vi "lp-server-timeouts.vi"() -> ()   [LabVIEW 2014]
uses:
  lvnanomsg/nanomsg_context.lvclass
  lvnanomsg/nanomsg_socket.lvclass
panel:
  in  "stop?":bool
  out "loop":i32
  in  "timeout":u32=500
  in  "endpoint":string="tcp://127.0.0.1:5555"
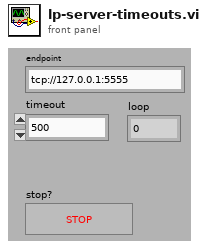
[diagram p1: front panel]
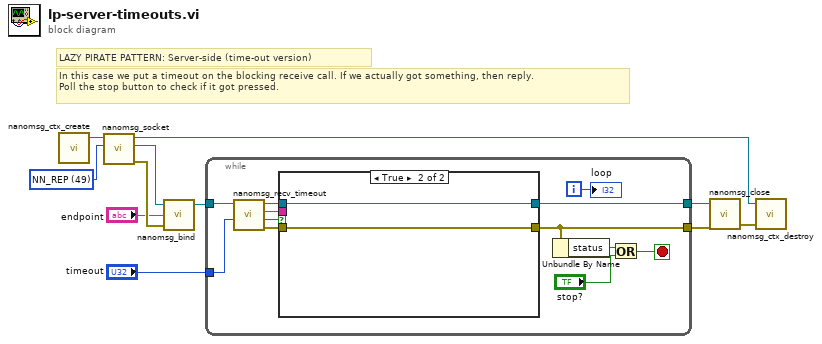
[diagram p0: block diagram]
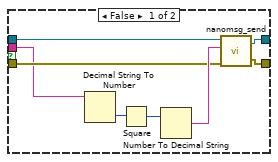
[diagram p2: hidden frame]
diagram:
  w7 = 49 items=["NN_WS"=-4, "NN_TCP"=-3, "NN_IPC"=-2, "NN_INPROC"=-1, "NN_SOL_SOCKET"=0, "NN_PAIR"=16, "NN_PUB"=32, "NN_SUB"=33, "NN_REQ"=48, "NN_REP"=49, "NN_PUSH"=80, "NN_PULL"=81, "NN_SURVEYOR"=98, "NN_RESPONDENT"=99, "NN_BUS"=112] ("socket type")
  # "In this case we put a timeout on the blocking receive call. If we actually got something, then reply.\nPoll the stop button to check if it got pressed."
  # "LAZY PIRATE PATTERN: Server-side (time-out version)"
  n1 = call "nanomsg_ctx_create.vi"() -> ("context out"=w6:refnum<class "nanomsg_context.lvclass">)  [unwired: 4 in, 1 out]
  n2 = call "nanomsg_socket.vi"("socket type"=w7, "context in"=w6) -> ("error out"=w10:errorcluster, "socket out"=w2:refnum<class "nanomsg_socket.lvclass">, "context out"=w1:refnum<class "nanomsg_context.lvclass">)  [unwired: 3 in]
  n3 = call "nanomsg_bind.vi"("error in"=w10, "endpoint"="endpoint", "socket in"=w2) -> ("socket out"=w8:refnum<class "nanomsg_socket.lvclass">)  [unwired: 1 in, 1 out]
  n4 = while {
    tunnel: "timeout" -> [w21]
    tunnel: w8 -> [w23]
    tunnel: [w17] -> w5
    tunnel: [w16] -> w3
    i -> [w19]
    stop <- w13 stop-if-true
    n5 = call "nanomsg_recv_timeout.vi"("timeout (ms)"=w21, "socket in"=w23) -> ("error out"=w18:errorcluster, "timeout?"=w12:bool, "part"=w20:string, "socket out"=w22:refnum<class "nanomsg_socket.lvclass">)  [unwired: 2 in]
    n6 = case shown="True" w12 {
      tunnel: w22 -> [w31 w33]
      tunnel: w20 -> [w24 _]
      tunnel: w18 -> [w27 w32]
      tunnel: [w26 w33] -> w17
      tunnel: [w25 w32] -> w16
      frame False {
        n7 = Decimal String To Number(string=w24) -> (number=w30:i32)  [unwired: 2 in, 1 out]
        n8 = Square(x=w30) -> (x^2=w29:i32)
        n9 = Number To Decimal String(number=w29) -> (decimal integer string=w28:string)  [unwired: 1 in]
        n10 = call "nanomsg_send.vi"("error in"=w27, "data"=w28, "socket in"=w31) -> ("error out"=w25:errorcluster, "socket out"=w26:refnum<class "nanomsg_socket.lvclass">)  [unwired: 1 in]
      }
      frame True {
      }
    }
    n11 = Unbundle By Name(w16) -> ("status"=w15:bool)
    n12 = Or(x=w15, y="stop?") -> (x .or. y?=w13:bool)
    "loop" <- w19
  }
  n13 = call "nanomsg_close.vi"("error in"=w3, "socket"=w5) -> ("error out"=w4:errorcluster)  [unwired: 3 in]
  n14 = call "nanomsg_ctx_destroy.vi"("error in"=w4, "context in"=w1) -> ()  [unwired: 3 in, 1 out]
